vi "PRIME Detector Wait for Command to Complete.vi"(5 "Observation":T2={"Priority"=0, "ID"="", "Observer"="", "Obj Name"="", "Obj Type"="", "RA and DEC String"={"RA"="HH:MM:SS.nnn", "DEC"="DEG:arcmin:arcsec.nn"}, "Filter Wheel 1"="", "Filter Wheel 2"="", "Integration Time"=0.0, "Observation Status"=enum."Error", "Offsets"={"RA"=0.0, "DEC"=0.0, "ROT"=0.0}, "Images"=0, "Dither Options"={"Dither"=enum."None", "Dither Radius"=0.0, "Dither Points"=0, "Dither Phase"=0.0}, "Comment 1"="", "Comment 2"=""}, 7 "Detector Config":T7={"Detector"=0, "Offsets"=[[0, 0, 0, 0, 0, 0, 0, 0, 0, 0, 0, 0, 0, 0, 0, 0, 0, 0, 0, 0, 0, 0, 0, 0, 0, 0, 0, 0, 0, 0, 0, 0]], "Detector Computer"={"Machine"="192.168.121.11", "Password"="rSL!nux23456", "FITS File Path"="", "Port"=44444, "Header Path"="", "Name"=""}, "FITS hdr template0"=path "", "FITS hdr template1"=path "", "FITS Data File Path"=path "", "FITS Detector Settings"={"Exp Time Short"=0.0, "# of Frames"=0.0, "Exp Time Long"=0.0, "# of Groups"=0.0, "Object Name"="", "Object"="", "Obs Type"="", "Image Type"="", "Observer"="", "Observer Affiliation"=""}, "Sim Folder"=path "", "Integration Mode"=enum."SSR", "Integration Time"=0.0, "Frame Int Time"=0.0} {"Offsets" format="%04x"; "Detector" items=["0", "1", "2"]}, 8 "error in (no error)":errorcluster, 9 "Exp Time":dbl=60.0, 10 "timeout (120s)":dbl=120.0, 11 "connection ID":refnum<k5>) -> (0 "error out":errorcluster, 1 "Image Map":map{string, T1}(c390), 2 "Status":T12, 3 "connection ID out":refnum<k5>)   [LabVIEW 2024, in "PRIME Detector.lvclass"]
uses:
  PRIME Detector.lvclass
  PRIME Detector cluster Status.ctl
  RIMAS Detector Config.ctl
  RIMAS Detector Server Config.ctl
  RIMAS Observation Config.ctl
  Detector enum Detector Integration Mode.ctl
  typedefs/CC cluster Observation.ctl
  Observation Queue/CC enum Observation Status.ctl
  Telescope/CC cluster Telescope Offsets.ctl
  typedefs/CC cluster Observation Dither Options.ctl
  typedefs/CC enum Dither Selection.ctl
  Detector Image typedef cluster.ctl
  Detector Class.lvclass
panel:
  in  "Image List":T11
  out "Time Remaining":dbl(knob) scale=-1.0..10.0
  out "Command":string
  # "sec"
  # "sec"
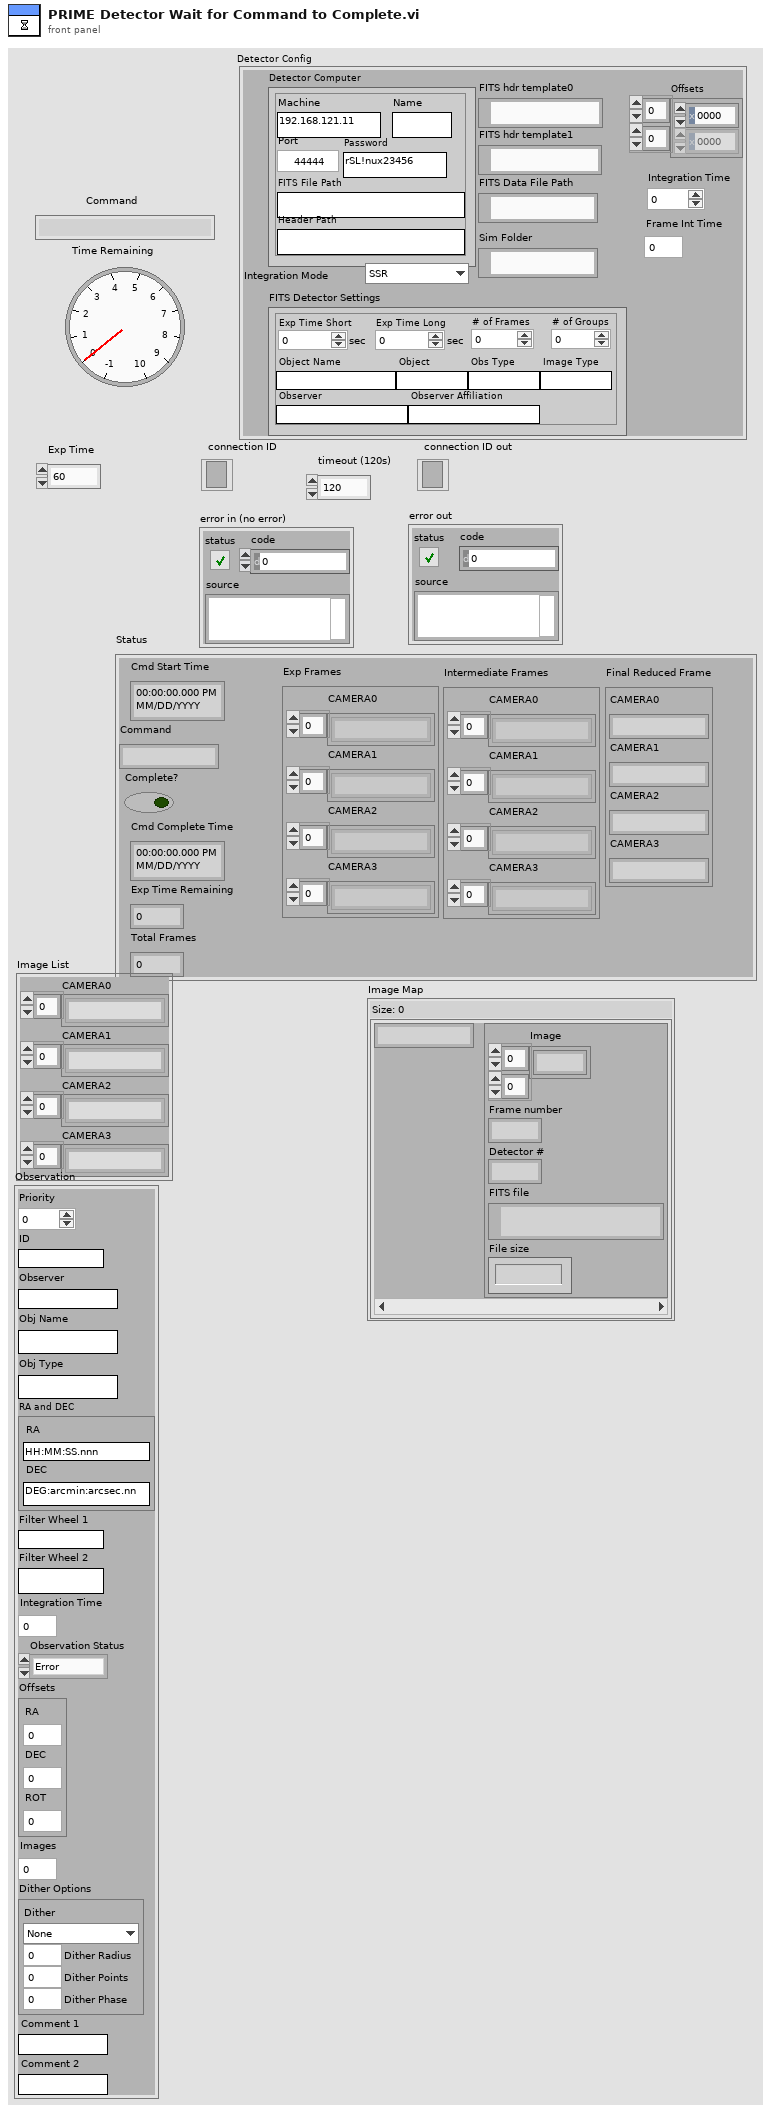
[diagram p1: front panel]
types:
  T1 = typedef "Detector Class.lvclass/Detector Image typedef cluster.ctl" = cluster{"Image":sgl[][], "Frame number":i32, "Detector #":u16, "FITS file":path, "File size":i64}
  T2 = typedef "CC cluster Observation.ctl" = cluster{"Priority":i32, "ID":string, "Observer":string, "Obj Name":string, "Obj Type":string, "RA and DEC String":cluster{"RA":string, "DEC":string}, "Filter Wheel 1":string, "Filter Wheel 2":string, "Integration Time":dbl, "Observation Status":T3, "Offsets":T4, "Images":i32, "Dither Options":T5, "Comment 1":string, "Comment 2":string}
  T3 = typedef "CC enum Observation Status.ctl" = enum16{"Ready", "Running", "Done", "Error"}
  T4 = typedef "CC cluster Telescope Offsets.ctl" = cluster{"RA":dbl, "DEC":dbl, "ROT":dbl}
  T5 = typedef "CC cluster Observation Dither Options.ctl" = cluster{"Dither":T6, "Dither Radius":dbl, "Dither Points":i32, "Dither Phase":dbl}
  T6 = typedef "CC enum Dither Selection.ctl" = enum16{"None", "Circle", "Random"}
  T7 = typedef "RIMAS Detector Config.ctl" = cluster{"Detector":u16, "Offsets":u16[][], "Detector Computer":T8, "FITS hdr template0":path, "FITS hdr template1":path, "FITS Data File Path":path, "FITS Detector Settings":T9, "Sim Folder":path, "Integration Mode":T10, "Integration Time":dbl, "Frame Int Time":dbl}
  T8 = typedef "RIMAS Detector Server Config.ctl" = cluster{"Machine":string, "Password":string, "FITS File Path":string, "Port":u16, "Header Path":string, "Name":string}
  T9 = typedef "RIMAS Observation Config.ctl" = cluster{"Exp Time Short":dbl, "# of Frames":dbl, "Exp Time Long":dbl, "# of Groups":dbl, "Object Name":string, "Object":string, "Obs Type":string, "Image Type":string, "Observer":string, "Observer Affiliation":string}
  T10 = typedef "Detector enum Detector Integration Mode.ctl" = enum16{"SSR", "CDS", "MEAN", "MEDIAN", "MODE", "MIIN", "MAX"}
  T11 = cluster{"CAMERA0":string[], "CAMERA1":string[], "CAMERA2":string[], "CAMERA3":string[]}
  T12 = typedef "PRIME Detector cluster Status.ctl" = cluster{"Cmd Start Time":timestamp, "Command":string, "Complete?":bool, "Cmd Complete Time":timestamp, "Exp Time Remaining":dbl, "Total Frames":i32, "Exp Frames":cluster{"CAMERA0":string[], "CAMERA1":string[], "CAMERA2":string[], "CAMERA3":string[]}, "Intermediate Frames":cluster{"CAMERA0":string[], "CAMERA1":string[], "CAMERA2":string[], "CAMERA3":string[]}, "Final Reduced Frame":cluster{"CAMERA0":string, "CAMERA1":string, "CAMERA2":string, "CAMERA3":string}}
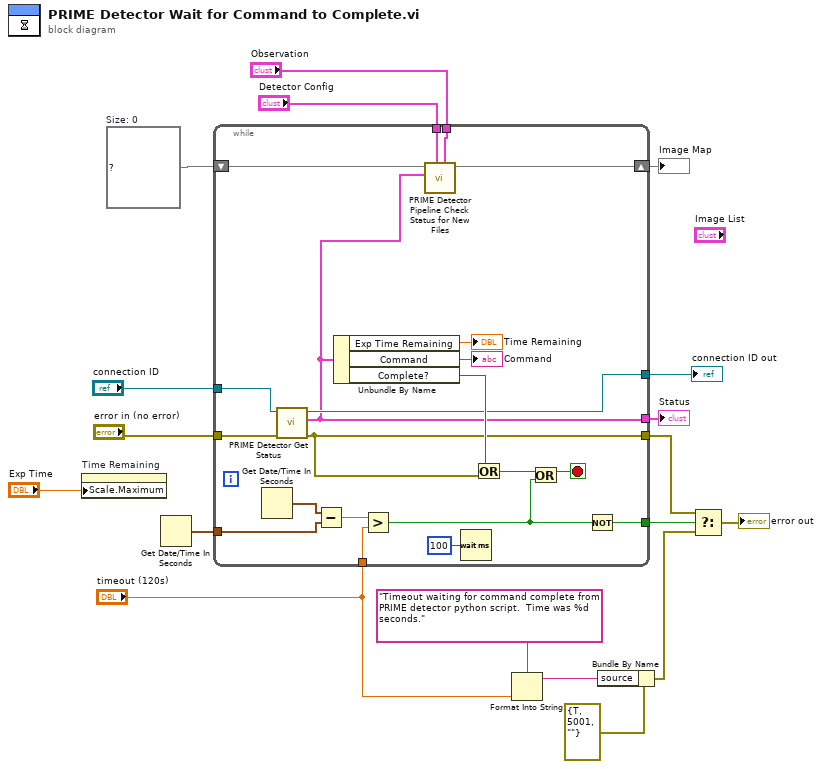
[diagram p0: block diagram]
diagram:
  w4 = map{string, T1} {}  # Size: 0
  n1 = property on="Time Remaining" class="Knob (strict)"("Scale.Maximum"="Exp Time") -> ()  [unwired: 2 in, 2 out]
  n2 = Get Date/Time In Seconds() -> (seconds since 1Jan1904=w16:timestamp)
  n3 = while {
    tunnel: "error in (no error)" -> [w39]
    tunnel: "connection ID" -> [w38]
    tunnel: [w35] -> w11
    tunnel: w16 -> [w32]
    tunnel: "timeout (120s)" -> [w30]
    tunnel: [w27] -> w14
    tunnel: [w21] -> w13
    tunnel: [w24] -> w12
    shift-right: [w22] -> w1
    shift-left: w4 -> [w23]
    tunnel: "Detector Config" -> [w20]
    tunnel: "Observation" -> [w19]
    stop <- w26 stop-if-true
    n4 = Get Date/Time In Seconds() -> (seconds since 1Jan1904=w33:timestamp)
    n5 = call "PRIME Detector Get Status.vi"("error in (no error)"=w39, "connection ID"=w38) -> ("error out"=w35:errorcluster, "Status"=w21:T12, "connection ID out"=w27:refnum<k5>)  [unwired: 6 in, 1 out]
    n6 = Subtract(x=w33, y=w32) -> (x-y=w31:dbl)
    n7 = Unbundle By Name(w21) -> ("Exp Time Remaining"=→"Time Remaining":dbl, "Command"=→"Command":string, "Complete?"=w37:bool)
    n8 = Greater?(x=w31, y=w30) -> (0:w25:bool)
    n9 = call "PRIME Detector Pipeline Check Status for New Files.vi"("Observation"=w19, "Detector Config"=w20, "Status"=w21, "Map in"=w23) -> ("Map out"=w22:map{string, T1})  [unwired: 6 in, 1 out]
    n10 = Wait (ms)(milliseconds to wait=u32 100 ("millisecond multiple")) -> ()  [unwired: 1 out]
    n11 = Or(x=w37, y=w35) -> (x .or. y?=w36:bool)
    n12 = Or(x=w36, y=w25) -> (x .or. y?=w26:bool)
    n13 = Not(x=w25) -> (.not. x?=w24:bool)
  }
  "connection ID out" <- w14
  "Status" <- w13
  "Image Map" <- w1
  n14 = Format Into String(format string="Timeout waiting for command complete from PRIME detector python script.  Time was %d seconds." ("source"), "timeout (120s)") -> (resulting string=w6:string)  [unwired: 2 in, 1 out]
  n15 = Bundle By Name(cluster=errorcluster {"status"=TRUE, "code"=5001, "source"=""} ("f"), "source"=w6) -> (w5:errorcluster)
  n16 = Select(t=w11, s=w12, f=w5) -> (s? t:f=→"error out":errorcluster)
